vi "机柜通讯test.vi"() -> ()   [LabVIEW 2015]
panel:
  out "消息":string
  in  "stop":bool
  in  "确定按钮":bool
  # "日志在\nD:\\testlog.txt\n使用说明：\n点击左上角白色箭头运行程序\n然后点击“切换开关”按钮\n消息栏显示128路测试信息\n测试完成后，不关闭程序，放置一段时间，再点击“切换开关”按钮。看连接是否断开。"
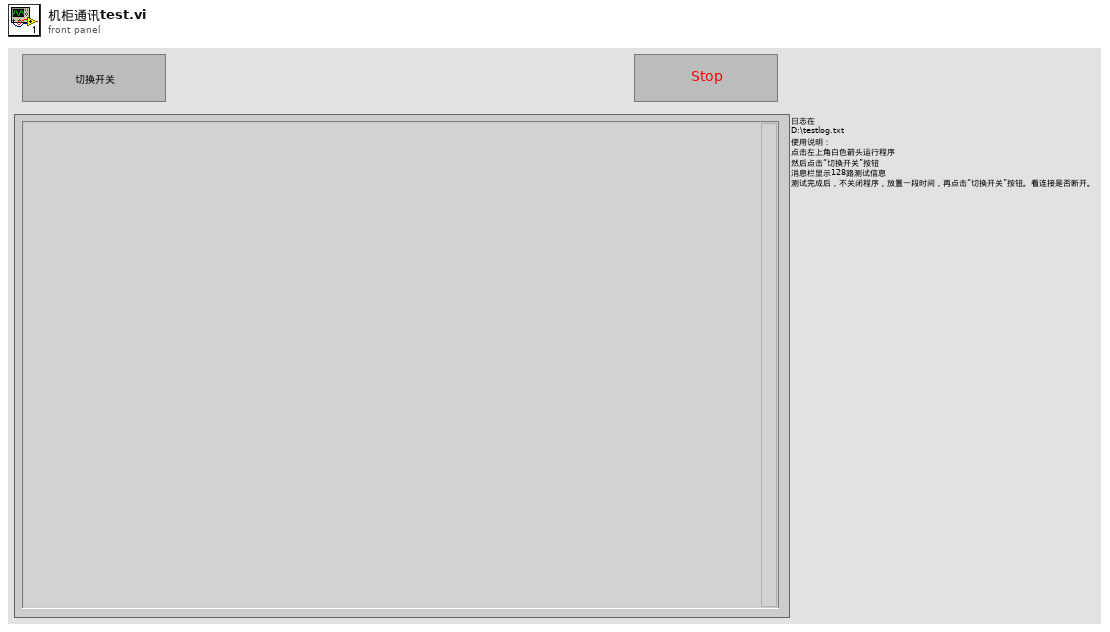
[diagram p1: front panel]
types:
  T1 = enum16{"open", "replace", "create", "open or create", "replace or create", "replace or create with confirmation"}
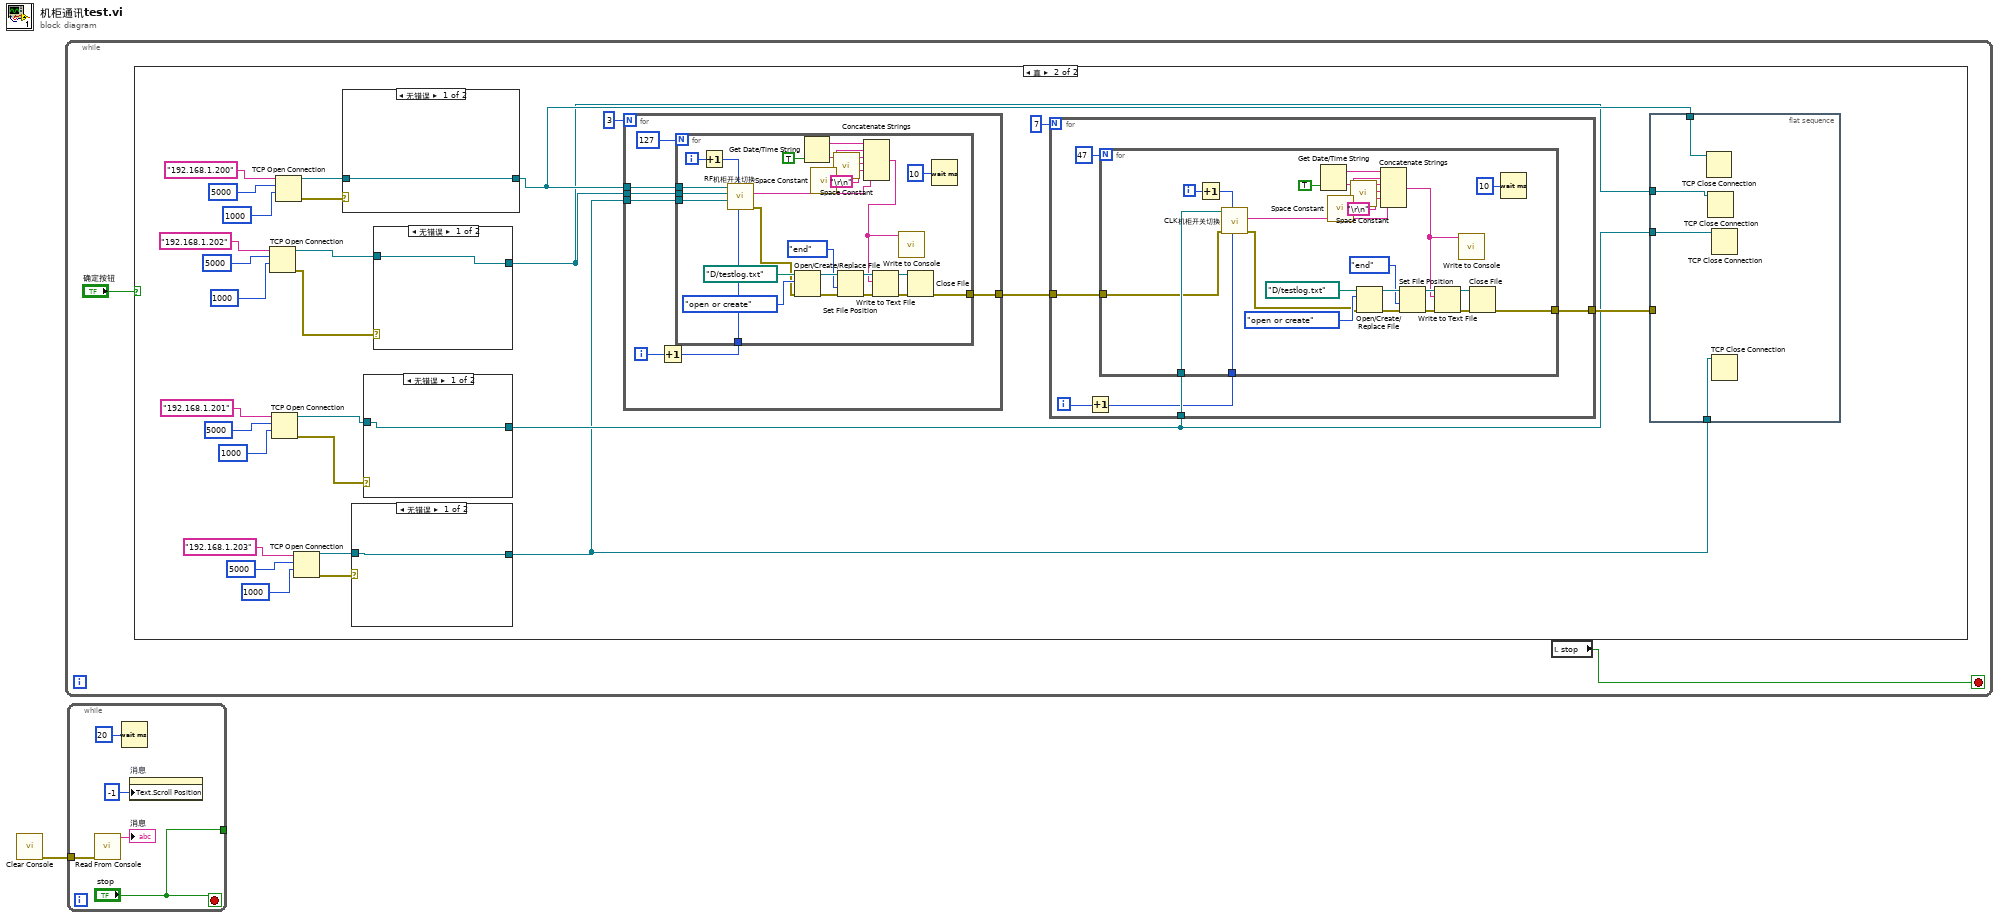
[diagram p0: block diagram]
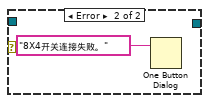
[diagram p3: hidden frame]
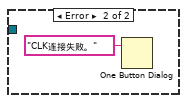
[diagram p4: hidden frame]
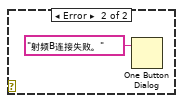
[diagram p5: hidden frame]
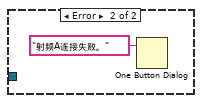
[diagram p6: hidden frame]
diagram:
  n1 = call "Clear Console.vi"() -> ("error out"=w1:errorcluster)  [unwired: 11 in]
  n2 = while {
    stop <- w2 stop-if-true
    n3 = case shown="真" "确定按钮" {
      frame False {
      }
      frame True {
        n4 = TCP Open Connection(address="192.168.1.202" ("IP(RF2)"), remote port or service name=u16 5000 ("PORT(RF)"), timeout ms (60000)=u16 1000 ("PORT(RF)")) -> (connection ID=w23:refnum<k5>, error out=w22:errorcluster)  [unwired: 2 in]
        n5 = TCP Open Connection(address="192.168.1.201" ("IP(RF2)"), remote port or service name=u16 5000 ("PORT(RF)"), timeout ms (60000)=u16 1000 ("PORT(RF)")) -> (connection ID=w18:refnum<k5>, error out=w17:errorcluster)  [unwired: 2 in]
        n6 = TCP Open Connection(address="192.168.1.200" ("IP(RF2)"), remote port or service name=u16 5000 ("PORT(RF)"), timeout ms (60000)=u16 1000 ("PORT(RF)")) -> (connection ID=w28:refnum<k5>, error out=w27:errorcluster)  [unwired: 2 in]
        n7 = TCP Open Connection(address="192.168.1.203" ("IP(RF2)"), remote port or service name=u16 5000 ("PORT(RF)"), timeout ms (60000)=u16 1000 ("PORT(RF)")) -> (connection ID=w13:refnum<k5>, error out=w12:errorcluster)  [unwired: 2 in]
        n8 = case shown="无错误" w27 {
          tunnel: [w42 _] -> w7
          tunnel: w28 -> [w42 _]
          frame No Error {
          }
          frame Error {
            n9 = One Button Dialog(message="射频A连接失败。") -> ()  [unwired: 1 in, 1 out]
          }
        }
        n10 = case shown="无错误" w12 {
          tunnel: w13 -> [w36 _]
          tunnel: [w36 _] -> w4
          frame No Error {
          }
          frame Error {
            n11 = One Button Dialog(message="8X4开关连接失败。") -> ()  [unwired: 1 in, 1 out]
          }
        }
        n12 = case shown="无错误" w17 {
          tunnel: w18 -> [w38 _]
          tunnel: [w38 _] -> w5
          frame No Error {
          }
          frame Error {
            n13 = One Button Dialog(message="CLK连接失败。") -> ()  [unwired: 1 in, 1 out]
          }
        }
        n14 = case shown="无错误" w22 {
          tunnel: [w40 _] -> w6
          tunnel: w23 -> [w40 _]
          frame No Error {
          }
          frame Error {
            n15 = One Button Dialog(message="射频B连接失败。") -> ()  [unwired: 1 in, 1 out]
          }
        }
        n16 = for {
          N: 3 -> [_]
          tunnel: w7 -> [w81]
          tunnel: w6 -> [w80]
          tunnel: w4 -> [w79]
          tunnel: [w75] -> w30
          i -> [w78]
          n17 = Increment(x=w78) -> (x+1=w77:i32)
          n18 = for {
            N: 127 -> [_]
            tunnel: w81 -> [w107]
            tunnel: w80 -> [w106]
            tunnel: w79 -> [w105]
            tunnel: w77 -> [w102]
            tunnel: [w91] -> w75
            i -> [w104]
            n19 = Increment(x=w104) -> (x+1=w103:i32)
            n20 = call "RF机柜开关切换.vi"("COM"=w102, "A"=w103, "8x4"=w105, "RF-B"=w106, "RF-A"=w107) -> ("error out"=w90:errorcluster, "ask"=w83:string)  [unwired: 5 in]
            n21 = Open/Create/Replace File(file path (use dialog)=path "D:/testlog.txt" ("文件（使用对话框）"), error in=w90, operation (0:open)=T1."open or create" ("操作(0:open)")) -> (refnum out=w98:refnum<file>, error out=w99:errorcluster)  [unwired: 3 in, 1 out]
            n22 = Get Date/Time String(want seconds? (F)=TRUE ("需要秒？(F)")) -> (date string=w88:string, time string=w87:string)  [unwired: 2 in]
            n23 = call <vilib>:"Space Constant.vi"() -> ("String"=w86:string)
            n24 = call <vilib>:"Space Constant.vi"() -> ("String"=w85:string)
            n25 = Set File Position(refnum=w98, from (0:start)=enum16{"start", "end", "current"}."end" ("自（0:起始）"), error in=w99) -> (refnum out=w100:refnum<file>, error out=w101:errorcluster)  [unwired: 1 in]
            n26 = Concatenate Strings(w88, w86, w87, w85, "\r\n", w83) -> (w82:string)
            n27 = Write to Text File(file (use dialog)=w100, text=w82, error in=w101) -> (refnum out=w96:refnum<file>, error out=w95:errorcluster)  [unwired: 1 in, 1 out]
            n28 = call "Write to Console.vi"("Input"=w82) -> ()  [unwired: 10 in, 1 out]
            n29 = Close File(refnum=w96, error in=w95) -> (error out=w91:errorcluster)  [unwired: 1 out]
            n30 = Wait (ms)(milliseconds to wait=u32 10 ("等待时间（毫秒）")) -> ()  [unwired: 1 out]
          }
        }
        n31 = for {
          N: 7 -> [_]
          tunnel: w5 -> [w49]
          tunnel: w30 -> [w48]
          tunnel: [w44] -> w8
          i -> [w47]
          n32 = Increment(x=w47) -> (x+1=w45:i32)
          n33 = for {
            N: 47 -> [_]
            tunnel: w49 -> [w74]
            tunnel: w48 -> [w73]
            tunnel: w45 -> [w72]
            tunnel: [w50] -> w44
            i -> [w71]
            n34 = Increment(x=w71) -> (x+1=w51:i32)
            n35 = call "CLK机柜开关切换.vi"("OUT"=w72, "IN"=w51, "error in"=w73, "CLK"=w74) -> ("error out"=w61:errorcluster, "ask"=w53:string)  [unwired: 6 in]
            n36 = Get Date/Time String(want seconds? (F)=TRUE ("需要秒？(F)")) -> (date string=w58:string, time string=w57:string)  [unwired: 2 in]
            n37 = call <vilib>:"Space Constant.vi"() -> ("String"=w56:string)
            n38 = call <vilib>:"Space Constant.vi"() -> ("String"=w55:string)
            n39 = Open/Create/Replace File(file path (use dialog)=path "D:/testlog.txt" ("文件（使用对话框）"), error in=w61, operation (0:open)=T1."open or create" ("操作(0:open)")) -> (refnum out=w67:refnum<file>, error out=w68:errorcluster)  [unwired: 3 in, 1 out]
            n40 = Concatenate Strings(w58, w56, w57, w55, "\r\n", w53) -> (w52:string)
            n41 = Set File Position(refnum=w67, from (0:start)=enum16{"start", "end", "current"}."end" ("自（0:起始）"), error in=w68) -> (refnum out=w69:refnum<file>, error out=w70:errorcluster)  [unwired: 1 in]
            n42 = Write to Text File(file (use dialog)=w69, text=w52, error in=w70) -> (refnum out=w65:refnum<file>, error out=w64:errorcluster)  [unwired: 1 in, 1 out]
            n43 = call "Write to Console.vi"("Input"=w52) -> ()  [unwired: 10 in, 1 out]
            n44 = Close File(refnum=w65, error in=w64) -> (error out=w50:errorcluster)  [unwired: 1 out]
            n45 = Wait (ms)(milliseconds to wait=u32 10 ("等待时间（毫秒）")) -> ()  [unwired: 1 out]
          }
        }
        n46 = flat-sequence {
          tunnel: w8 -> [_]
          tunnel: w7 -> [w35]
          tunnel: w6 -> [w34]
          tunnel: w5 -> [w33]
          tunnel: w4 -> [w32]
          frame #0 {
            n47 = TCP Close Connection(connection ID=w35) -> ()  [unwired: 2 in, 2 out]
            n48 = TCP Close Connection(connection ID=w34) -> ()  [unwired: 2 in, 2 out]
            n49 = TCP Close Connection(connection ID=w33) -> ()  [unwired: 2 in, 2 out]
            n50 = TCP Close Connection(connection ID=w32) -> ()  [unwired: 2 in, 2 out]
          }
        }
      }
    }
    n51 = local read "stop"() -> (w2:bool)
  }
  n52 = while {
    tunnel: w1 -> [w111]
    tunnel: ["stop"] -> _
    stop <- "stop" stop-if-true
    n53 = call "Read From Console.vi"("error in (no error)"=w111) -> ("Output"=→"消息":string)  [unwired: 9 in, 1 out]
    n54 = Wait (ms)(milliseconds to wait=u32 20) -> ()  [unwired: 1 out]
    n55 = property on="消息" class="Str"("Text.Scroll Position"=i8 -1 ("milliseconds to wait")) -> ()  [unwired: 2 in, 2 out]
  }
